vi "ActionVIOnLoad.vi"(8 "error in (no error)":errorcluster, 11 "Device Item Ref in":T1 format="%.0x") -> (0 "error out":errorcluster, 3 "Device Item Ref out":T1 format="%.0x")   [LabVIEW 2019, in "OPC UA Client Addon System Explorer.lvlib"]
uses:
  OPC UA Client Addon System Explorer.lvlib
  <vilib>/NI VeriStand/Custom Device API/Custom Device Item Ref.ctl
  NationalInstruments.VeriStand.SystemDefinitionAPI
  Addon Shared/SubVIs/Constants.vi
  Addon Shared/OPC UA Client Addon Shared.lvlib
  <vilib>/NI/NI VeriStand Advanced SysDef API/SysDef API/Advanced System Definition.lvlib
  <vilib>/NI VeriStand/Custom Device API/Custom Device API.lvlib
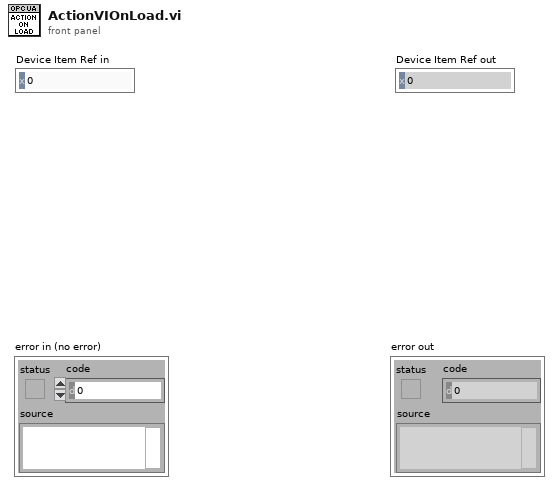
[diagram p1: front panel]
types:
  T1 = typedef "Custom Device API.lvlib/Custom Device Item Ref.ctl" = u64
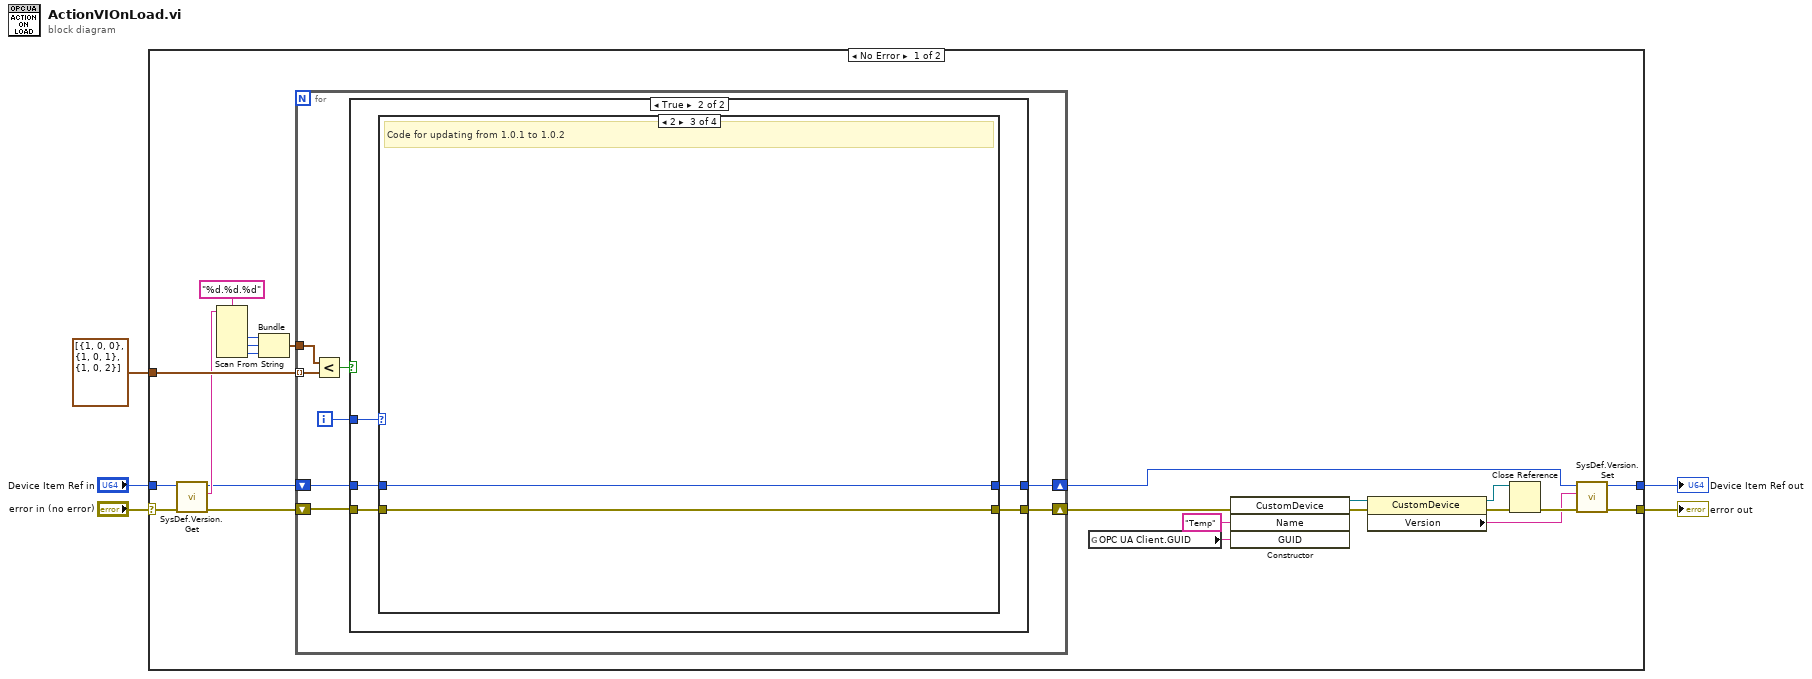
[diagram p0: block diagram]
diagram:
  n1 = case shown="No Error" "error in (no error)" {
    selector: "error in (no error)" -> [w11 w53]
    tunnel: [w21 w53] -> w2
    tunnel: "Device Item Ref in" -> [w10 w52]
    tunnel: [w20 w52] -> w1
    tunnel: cluster{i32, i32, i32}[] [{1, 0, 0}, {1, 0, 1}, {1, 0, 2}] -> [w28 _]
    frame No Error {
      n2 = call <vilib>:"SysDef.Version.Get.vi"("error in (no error)"=w11, "nodeID"=w10) -> ("error out"=w7:errorcluster, "Version"=w14:string, "nodeID out"=w6:u64)  [unwired: 7 in]
      n3 = Scan From String(format string="%d.%d.%d", input string=w14) -> (output 1=w13:i32, output 2=w12:i32, output 3=w15:i32)  [unwired: 5 in, 3 out]
      n4 = Bundle(w13, w12, w15) -> (w8:cluster{i32, i32, i32})  [unwired: 1 in]
      n5 = for {
        tunnel: w28 -> [w31] mode=indexing
        shift-right: [w35] -> w19
        shift-left: w7 -> [w29]
        shift-right: [w34] -> w18
        shift-left: w6 -> [w30]
        tunnel: w8 -> [w32]
        i -> [w33]
        n6 = Less?(x=w32, y=w31) -> (x < y?=w36:bool)
        n7 = case shown="True" w36 {
          tunnel: w29 -> [w38 w43]
          tunnel: [w38 w42] -> w35
          tunnel: w30 -> [w37 w39]
          tunnel: [w37 w40] -> w34
          tunnel: w33 -> [_ w41]
          frame False {
          }
          frame True {
            n8 = case shown="2" w41 {
              tunnel: w43 -> [w45 w47 w49 w51]
              tunnel: [w45 w47 w49 w51] -> w42
              tunnel: [w44 w46 w48 w50] -> w40
              tunnel: w39 -> [w44 w46 w48 w50]
              frame Default {
                # "Nothing to update"
              }
              frame 1 {
                # "Code for updating from 1.0.0 to 1.0.1"
              }
              frame 2 {
                # "Code for updating from 1.0.1 to 1.0.2"
              }
              frame 0 {
                # "Initial Onload"
              }
            }
          }
        }
      }
      n9 = global read "Constants.vi" "OPC UA Client.GUID"() -> (w16:string)
      n10 = constructor class="CustomDevice"(error in=w19, "Name"="Temp", "GUID"=w16) -> (reference out=w27:refnum<k24>, error out=w26:errorcluster)  [unwired: 2 in, 3 out]
      n11 = property class="CustomDevice"(reference=w27, error in=w26) -> (reference out=w24:refnum<k24>, error out=w25:errorcluster, "Version"=w22:string)
      n12 = Close Reference(reference=w24, error in (no error)=w25) -> (error out=w23:errorcluster)
      n13 = call <vilib>:"SysDef.Version.Set.vi"("error in (no error)"=w23, "Version"=w22, "nodeID"=w18) -> ("error out"=w21:errorcluster, "nodeID out"=w20:u64)  [unwired: 7 in]
    }
    frame Error {
    }
  }
  "error out" <- w2
  "Device Item Ref out" <- w1
